vi "LINC Get Packet Properties.vi"(8 "error in (no error)":errorcluster, 11 "control reference":refnum<vi>) -> (0 "error out":errorcluster, 2 "properties":cluster{"hazardous":bool})   [LabVIEW 2018, in "STEPkgDriver_LINC.lvlib"]
uses:
  STEPkgDriver_LINC.lvlib
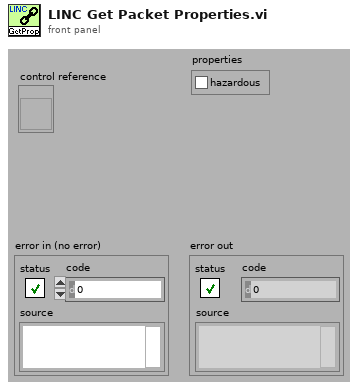
[diagram p1: front panel]
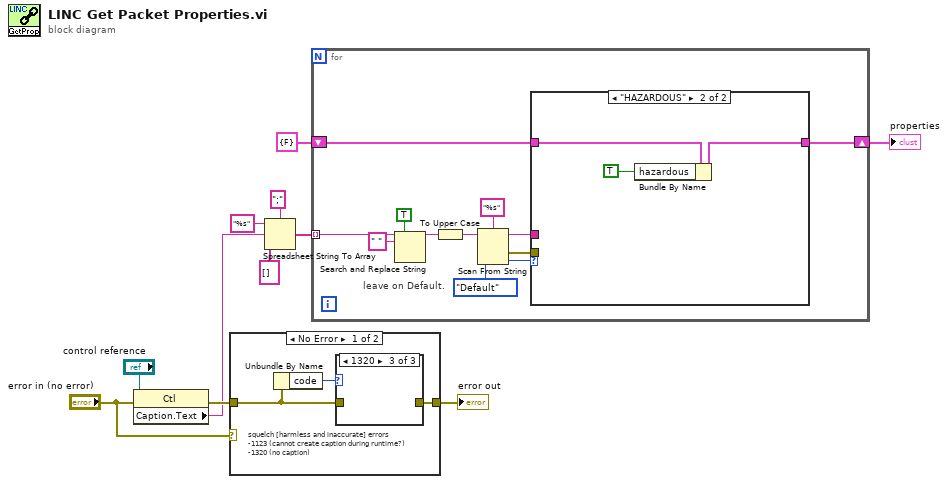
[diagram p0: block diagram]
diagram:
  n1 = property class="Ctl"(reference="control reference", error in="error in (no error)") -> (error out=w5:errorcluster, "Caption.Text"=w2:string)  [unwired: 1 out]
  n2 = case shown="No Error" "error in (no error)" {
    tunnel: [w13 w16] -> w1
    tunnel: w5 -> [w12 w16]
    frame No Error {
      # "squelch [harmless and inaccurate] errors\n-1123 (cannot create caption during runtime?)\n-1320 (no caption)"
      n3 = Unbundle By Name(w12) -> ("code"=w14:i32)
      n4 = case shown="1320" w14 {
        tunnel: w12 -> [w15 _ _]
        tunnel: [w15 _ _] -> w13
        frame Default {
        }
        frame 1123 {
        }
        frame 1320 {
        }
      }
    }
    frame Error {
    }
  }
  "error out" <- w1
  n5 = Spreadsheet String To Array(delimiter (Tab)=";", format string="%s", spreadsheet string=w2, array type (2D Dbl)=string[] []) -> (array=w8:string[])
  n6 = for {
    tunnel: w8 -> [w19] mode=indexing
    shift-right: [w17] -> w7
    shift-left: cluster{"hazardous":bool} {"hazardous"=FALSE} ("properties") -> [w18]
    # "leave on Default."
    n7 = Search and Replace String(replace all?=TRUE ("replace all? (F)"), input string=w19, search string=" ") -> (result string=w20:string)  [unwired: 5 in, 3 out]
    n8 = To Upper Case(1:w20) -> (0:w27:string)
    n9 = Scan From String(format string="%s", input string=w27, default 1=enum16{"Default", "HAZARDOUS"}."Default") -> (remaining string=w24:string, error out=w23:errorcluster, output 1=w25:enum16{"Default", "HAZARDOUS"})  [unwired: 2 in, 1 out]
    n10 = case shown="\"HAZARDOUS\"" w25 {
      tunnel: w24 -> [_ _]
      tunnel: w23 -> [_ _]
      tunnel: w18 -> [w29 w32]
      tunnel: [w29 w31] -> w17
      frame "Default" {
      }
      frame "HAZARDOUS" {
        n11 = Bundle By Name(cluster=w32, "hazardous"=TRUE ("ID")) -> (w31:cluster{"hazardous":bool})
      }
    }
  }
  "properties" <- w7
